vi "Build Target.vi"   [LabVIEW 2017, in "Scripts.lvlib"]
doc: "Builds all components and the VI package for a project/target.\n\nThis VI is called as part of the automated build process. It is configured to run when loaded."
uses:
  Scripts.lvlib
  <vilib>/AppBuilder/AB_API_Simple/Build (path).vi
  <vilib>/AppBuilder/AB_API_Simple/NI_App_Builder_API.lvlib
  <vilib>/JKI/VIPM API/VIPM API_vipm_api.lvlib
panel:
  # "Overview: Builds all components and the VI package for a project/target\nRequirements: Caraya, JKI State Machine, OpenG Array Library, OpenG File Library, VIPM Pro, VIPM API\nInstructions: Run this VI."
  # "This VI is called as part of the automated build process. It should not be aborted or closed while running. It will build all of the Source Distribution build specifications for the project/target, starts VIPM if it is not already running, builds the package, then closes LabVIEW. The VIPM is left running. This VI is configured to run when called.\n\nThis VI will fail if Caraya, JKI State Machine, OpenG Array Library, OpenG File Library, VIPM Pro, and the VIPM API are not installed for the target LabVIEW version, i.e. LabVIEW 2015."
types:
  T1 = typedef "VIPM API_vipm_api.lvlib/VI Package Build Spec Data Cluster_vipm_api.ctl" = cluster{"Package Version":T2, "Product Name":string, "Company Name":string, "Author Name (Person or Company)":string, "Product Homepage (URL)":string, "Legal Copyright":string, "License Agreement Name":string, "Product Description Summary":string, "Product Description":string, "Release Notes - Change Log":string}
  T2 = typedef "VIPM API_vipm_api.lvlib/Version Info Cluster_vipm_api.ctl" = cluster{"major":u32, "minor":u32, "patch":u32, "build":u32}
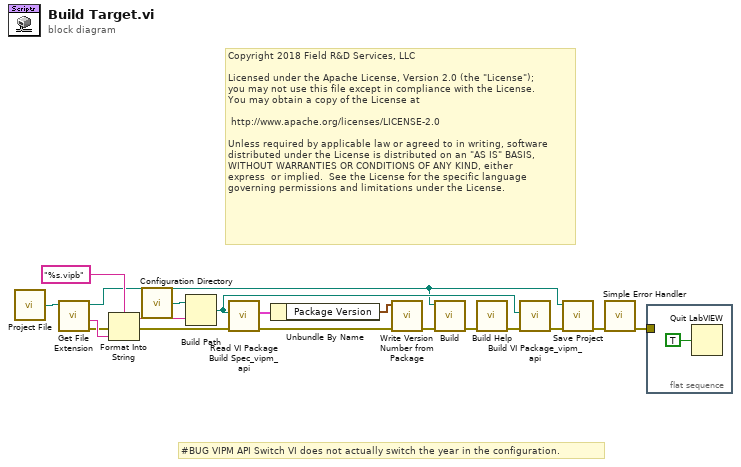
[diagram p0: block diagram]
diagram:
  # "Copyright 2018 Field R&D Services, LLC\n\nLicensed under the Apache License, Version 2.0 (the \"License\");\nyou may not use this file except in compliance with the License.\nYou may obtain a copy of the License at\n\n\thttp://www.apache.org/licenses/LICENSE-2.0\n\nUnless required by applicable law or agreed to in writing, software\ndistributed under the License is distributed on an \"AS IS\" BASIS,\nWITHOUT WARRANTIES OR CONDITIONS OF ANY KIND, either \nexpress  or implied.  See the License for the specific language \ngoverning permissions and limitations under the License."
  # "#BUG VIPM API Switch VI does not actually switch the year in the configuration."
  n1 = call "Project File.vi"() -> ("Project File"=w13:path)
  n2 = call <vilib>:"Get File Extension.vi"("file"=w13) -> ("error out"=w11:errorcluster, "filename without extension"=w18:string, "dup file"=w2:path)  [unwired: 6 in, 2 out]
  n3 = Format Into String(format string="%s.vipb", error in=w11, w18) -> (resulting string=w16:string, error out=w10:errorcluster)  [unwired: 1 in]
  n4 = call "Configuration Directory.vi"() -> ("Configuration Directory"=w14:path)
  n5 = Build Path(base path=w14, name or relative path=w16) -> (appended path=w9:path)
  n6 = call <vilib>:"Read VI Package Build Spec_vipm_api.vi"("error in (no error)"=w10, "Path to VIPB File"=w9) -> ("error out"=w8:errorcluster, "VI Package Build Spec Data"=w6:T1)  [unwired: 8 in]
  n7 = Unbundle By Name(w6) -> ("Package Version"=w5:T2)
  n8 = call "Write Version Number from Package.vi"("Error In"=w8, "Package Version"=w5) -> ("Error Out"=w7:errorcluster)  [unwired: 9 in]
  n9 = call-poly <vilib>:"Build.vi"("error in (no error)"=w7, "Path to project"=w2) -> ("error out"=w4:errorcluster)  [unwired: 8 in, 1 out]
  n10 = call "Build Help.vi"("Error In"=w4) -> ("Error Out"=w3:errorcluster)  [unwired: 9 in, 1 out]
  n11 = call <vilib>:"Build VI Package_vipm_api.vi"("error in (no error)"=w3, "Path to VIPB File"=w9) -> ("error out"=w12:errorcluster)  [unwired: 8 in, 1 out]
  n12 = call "Save Project.vi"("Error In"=w12, "Proejct In"=w2) -> ("Error Out"=w1:errorcluster)  [unwired: 8 in, 1 out]
  n13 = call <vilib>:"Simple Error Handler.vi"("error in (no error)"=w1) -> ("error out"=w15:errorcluster)  [unwired: 4 in, 4 out]
  n14 = flat-sequence {
    tunnel: w15 -> [_]
    frame #0 {
      n15 = Quit LabVIEW(quit? (T)=TRUE) -> ()
    }
  }
